vi "Rd Wr settings jsonfile counter.vi"(8 "error in (no error)":errorcluster, 9 "Settings File":string="CC File Counter.json", 10 "Write? (F:Read)":bool, 11 "FileCounter":T1) -> (0 "error out":errorcluster, 3 "FileCounter":T1)   [LabVIEW 2021]
uses:
  PRIME cluster File Counter.ctl
  2e80df6d-94aa-46b9-8b94-ceea8c057880.vi
  659fb017-0e9f-42f9-b06e-930303f00cbc.vi
  <vilib>/JDP Science/JSONtext/Find Item.vi
  <vilib>/JDP Science/JSONtext/Next JSON Value.vi
  <vilib>/JDP Science/JSONtext/String Subset.vi
  <vilib>/JDP Science/JSONtext/Parsing/Advance past next JSON Value (inlined COPY).vi
  <vilib>/JDP Science/JSONtext/Parsing/Advance past whitespace.vi
  <vilib>/JDP Science/JSONtext/Parsing/Advance past String.vi
  <vilib>/JDP Science/JSONtext/Parsing/Advance past Number.vi
  <vilib>/JDP Science/JSONtext/Parsing/Advance past Line Ending.vi
  <vilib>/JDP Science/JSONtext/Parsing/Parse Full Path or Item Name.vi
  <vilib>/JDP Science/JSONtext/Parsing/Advance past Array.vi
  <vilib>/JDP Science/JSONtext/Parsing/Advance past Object.vi
  <vilib>/JDP Science/JSONtext/support/Error Cluster From Code.vi
  <vilib>/JDP Science/JSONtext/Offset/Find Item Locations by Path.vi
  <vilib>/JDP Science/JSONtext/JSON text to Variant.vi
  <vilib>/JDP Science/JSONtext/Variant to JSON Text.vi
  <vilib>/JDP Science/JSONtext/Set Item.vi
  <vilib>/JDP Science/JSONtext/LVClass Serializer/JSONtext LVClass Serializer.lvclass
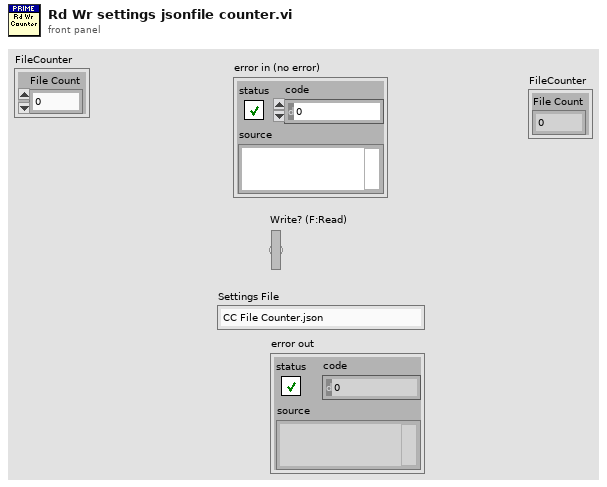
[diagram p1: front panel]
types:
  T1 = typedef "PRIME cluster File Counter.ctl" = cluster{"File Count":i32}
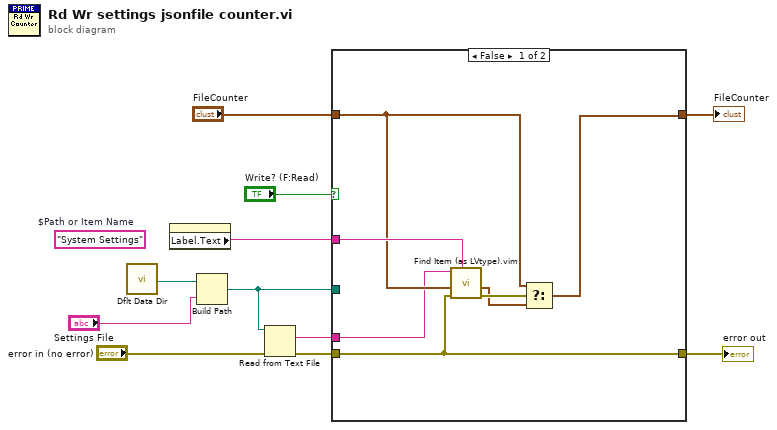
[diagram p0: block diagram]
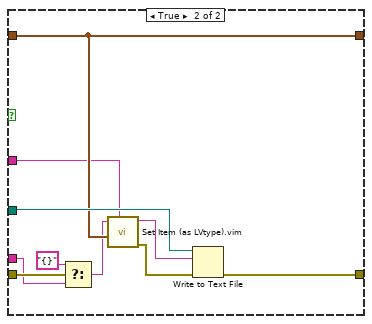
[diagram p2: hidden frame]
diagram:
  (unwired) "System Settings"  # $Path or Item Name
  n1 = call <vilib>:"Dflt Data Dir.vi"() -> ("App:Default Data Directory"=w8:path)
  n2 = property class="Clust (strict)"() -> ("Label.Text"=w1:string)  [unwired: 2 in, 2 out]
  n3 = Build Path(base path=w8, name or relative path="Settings File") -> (appended path=w2:path)
  n4 = Read from Text File(file (use dialog)=w2, error in="error in (no error)") -> (text=w3:string, error out=w4:errorcluster)  [unwired: 2 in, 2 out]
  n5 = case shown="False" "Write? (F:Read)" {
    tunnel: w4 -> [w12 w23]
    tunnel: "FileCounter" -> [w16 w26]
    tunnel: w2 -> [_ w28]
    tunnel: [w12 w27] -> w7
    tunnel: [w18 w26] -> w6
    tunnel: w1 -> [w17 w25]
    tunnel: w3 -> [w13 w21]
    frame False {
      n6 = call "Find Item (as LVtype).vim"("$Path or Item Name"=w17, "error in (no error)"=w12, "Data Type and Default Value"=w16, "JSON"=w13) -> ("error out"=w15:errorcluster, "Data"=w14:T1)  [unwired: 4 in, 2 out]
      n7 = Select(t=w16, s=w15, f=w14) -> (s? t:f=w18:T1)
    }
    frame True {
      n8 = Select(t="{}" ("JSON"), s=w23, f=w21) -> (s? t:f=w20:string)
      n9 = call "Set Item (as LVtype).vim"("$Path or Item Name"=w25, "Anything"=w26, "JSON"=w20) -> ("error out"=w19:errorcluster, "<JSON>"=w24:string)  [unwired: 5 in, 1 out]
      n10 = Write to Text File(file (use dialog)=w28, text=w24, error in=w19) -> (error out=w27:errorcluster)  [unwired: 1 in, 2 out]
    }
  }
  "error out" <- w7
  "FileCounter" <- w6
